vi "Is Created Event.vi"(7 "jettl in":refnum<class "jettl.lvclass">, 9 "Created Event Alias":string, 10 "Queue Mailbox":refnum<data-value>) -> (2 "Is Created Event?":bool, 5 "jettl out":refnum<class "jettl.lvclass">)   [LabVIEW 2021, in "jettl.lvlib" / "Addresses.lvlib"]
uses:
  Addresses.lvlib
  jettl/jettl.lvclass
  Addresses/Addresses.lvclass
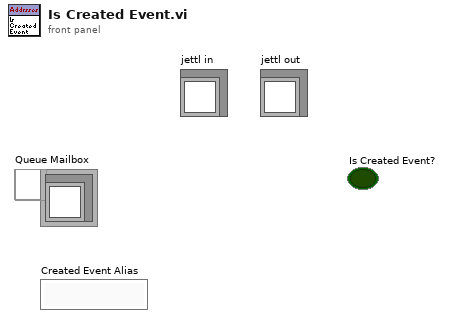
[diagram p1: front panel]
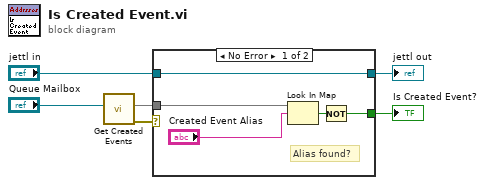
[diagram p0: block diagram]
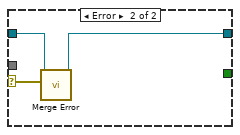
[diagram p2: hidden frame]
diagram:
  n1 = call "Get Created Events.vi"("Queue Mailbox"="Queue Mailbox") -> ("error out"=w1:errorcluster, "Created Events"=w2:map{string, refnum<data-value>})  [unwired: 9 in]
  n2 = case shown="No Error" w1 {
    selector: w1 -> [_ w12]
    tunnel: [w11 w13] -> w5
    tunnel: "jettl in" -> [w11 w14]
    tunnel: w2 -> [w8 _]
    tunnel: [w7 _] -> w4
    frame No Error {
      # "Alias found?"
      n3 = Look In Map(map=w8, key="Created Event Alias") -> (key not found?=w9:bool)  [unwired: 1 in, 1 out]
      n4 = Not(x=w9) -> (.not. x?=w7:bool)
    }
    frame Error {
      n5 = call-dynamic "Merge Error.vi"("Error"=w12, "Merge Error in"=w14) -> ("Merge Error out"=w13:refnum<class "jettl.lvclass">)  [unwired: 9 in]
    }
  }
  "jettl out" <- w5
  "Is Created Event?" <- w4
